vi "Strip_filename_fr_string.vi"(1 "Input String":string, 2 "y":i32) -> (0 "Output String":string)   [LabVIEW 2010]
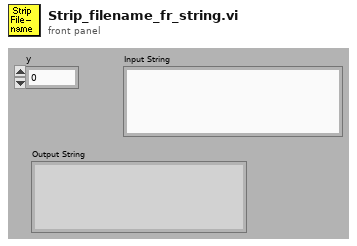
[diagram p1: front panel]
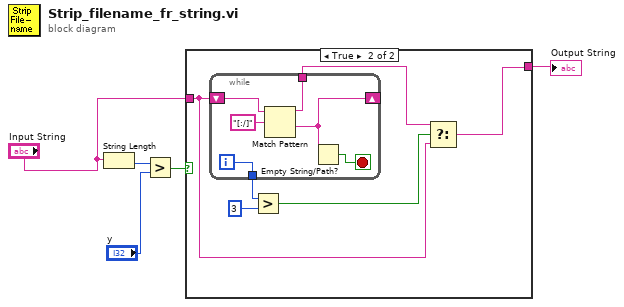
[diagram p0: block diagram]
diagram:
  n1 = String Length(string="Input String") -> (length=w2:i32)
  n2 = Greater?(x=w2, y="y") -> (0:w5:bool)
  n3 = case shown="True" w5 {
    tunnel: "Input String" -> [w6 w8]
    tunnel: [w6 w7] -> w1
    frame False {
    }
    frame True {
      n4 = while {
        shift-right: [w16] -> _
        shift-left: w8 -> [w17]
        tunnel: [w14] -> w9
        tunnel: [w13] -> w12
        i -> [w13]
        stop <- w15 stop-if-true
        n5 = Match Pattern(string=w17, regular expression="[:/]") -> (before substring=w14:string, after substring=w16:string)  [unwired: 3 out]
        n6 = Empty String/Path?(string/path=w16) -> (empty?=w15:bool)
      }
      n7 = Greater?(x=w12, y=3) -> (0:w10:bool)
      n8 = Select(t=w9, s=w10, f=w8) -> (s? t:f=w7:string)
    }
  }
  "Output String" <- w1
